vi "supermlo photo v3_LV2010 GFIREST VARIANT.vi"() -> ()   [LabVIEW 2010]
uses:
  <vilib>/Utility/file.llb/Read From Spreadsheet File (DBL).vi
  Instance          10 25Saved   supermlo photo v3 .vi
  Instance           9 25Saved   supermlo photo v3 .vi
  Instance           8 25Saved   supermlo photo v3 .vi
  Instance          15 25Saved   supermlo photo v3 .vi
  Instance          16 25Saved   supermlo photo v3 .vi
  Instance          17 25Saved   supermlo photo v3 .vi
  Instance          12 25Saved   supermlo photo v3 .vi
  Instance          13 25Saved   supermlo photo v3 .vi
  Instance          14 25Saved   supermlo photo v3 .vi
  <vilib>/Utility/file.llb/Write To Spreadsheet File (DBL).vi
panel:
  out "Lockin corrected counter graoh":cluster{"all rows":dbl[], "all rows":dbl[]}[](graph)
  in  "Lockin panel":T1={"slope"=1, "Input Mode"=0, "time constant"=6, "display type"=1, "Range"=7, "Line reject"=1, "Filter Type"=0, "Auto freq tuning"=TRUE, "Filter Frequency (Hz)"=1000.0, "Auto Sensitivity"=FALSE, "Auto Measure"=FALSE, "Auto Phase"=TRUE} {"Filter Frequency (Hz)" min=2.0 max=1250000.0 step=1.0; "Filter Type" items=["Flat", "Notch", "Low-Pass", "Bandpass"]; "Line reject" items=["OFF", "2F", "F", "F & 2F"]; "Range" items=["100 nV", "300 nV", "1 uV", "3 uV", "10 uV", "30 uV", "100 uV", "300 uV", "1 mV", "3 mV", "10 mV", "30 mV", "100 mV", "300 mV", "1 V", "3 V"]; "display type" items=["Output %", "Output calibrated ", "Ratio", "log Ratio", "ADC 1", "ADC 2", " ADC 3", "ADC 4", "Noise %", "Noise Calibrated", "Ref. Frequency"]; "time constant" items=["1 ms", "3 ms", "10 ms", "30 ms", "100 ms", "300 ms", "1 s", "3 s", "10 s", "30 s", "100 s", "300 s", "1 ks", "3 ks"]; "Input Mode" items=["Voltage Input ( A or A-B)", "Current Input 10E6 V/A", "Current Input 10E8 V/A"]; "slope" items=["6dB/octave", "12dB/octave"]}
  out "Wavelength Range Warning":bool
  out "wavelength":i32=692
  out "counter A":i32=70
  out "counter B":i32
  out "lockin":dbl=78.0 format="%.3e"
  out "Lockin Graph":cluster{"all rows":dbl[], "all rows":dbl[]}[](graph)
  out "Counter Graph":cluster{"all rows":dbl[], "all rows":dbl[]}[](graph)
  in  "GPIB Address Lock-In":u8=12 min=1 max=32 step=1
  in  "GPIB Address OSC (GPIB::4)":string="GPIB0::4"
  in  "Parallel Port Address":i16=888 format="%.0x"
  in  "Mode Control":T2(tab)=enum."Sweep 2"
  in  "Wavelength":dbl=500.0
  out "Waveform Graph":cluster{ext, ext, ext[]}(graph)
  in  "Pull Data From Oscilloscope":bool
  in  "waveform source (ch1:0)":i32(ring) items=["Channel 1", "Channel 2", "Channel 3", "Channel 4", "Reference 1", "Reference 2", "Reference 3", "Reference 4", "Math 1", "Math 2", "Math 3"]
  in  "Time For Scan (seconds)":dbl=30.0
  in  "Final Wavelength (scan)":dbl=425.0
  in  "Initial Wavelength (scan)":dbl=546.0
  out "XY Graph":cluster{"Y":dbl[], "Y":dbl[]}[](graph)=[{"Y"=[424.0, 425.0, 426.0, 427.0, 428.0, 429.0, 430.0, 431.0, 432.0, 433.0, 434.0], "Y"=[23.190000534057617, 23.65999984741211, 23.200000762939453, 22.600000381469727, 24.850000381469727, 24.90999984741211, 24.979999542236328, 24.940000534057617, 24.829999923706055, 24.860000610351562, 24.799999237060547]}]
  in  "Wait Time (s)":dbl=50.0
  in  "Step Size (nm)":dbl=1.0
  in  "Final Wavelength (sweep)":dbl=435.0
  in  "Initial Wavelength (sweep)":dbl=424.0
  in  "raster settings\nxV xHz yV yHz":string
  in  "note":string
  in  "532 power":string="0"
  in  "Green Filter in = 1":string="1"
  out "String":string
  in  "Wait Time (s) (sweep2)":dbl=5.0
  in  "Step Size (nm) (sweep2)":dbl=1.0
  in  "Final Wavelength (sweep2)":dbl=510.0
  in  "Initial Wavelength (sweep2)":dbl=420.0
  in  "Start Wavelength":dbl=430.0
  # "Oscilloscope Setup"
  # "Monochromator Setup"
  # "Lock-In Setup"
  # "GABE'S VARIANT, appends to TEMP rather than overwrites"
  # "LAST DATA POINT"
  # "Lockin Amplifier"
  # "SR400 photon counter:\n1. Run photon counter vi\nor manually control desired\nsettings.\n2. Set Wait Time to Tpreset\n3. Run this program.\nnote: # count periods N = 1"
  # "Note: set wait time to\nTpreset value on SR400"
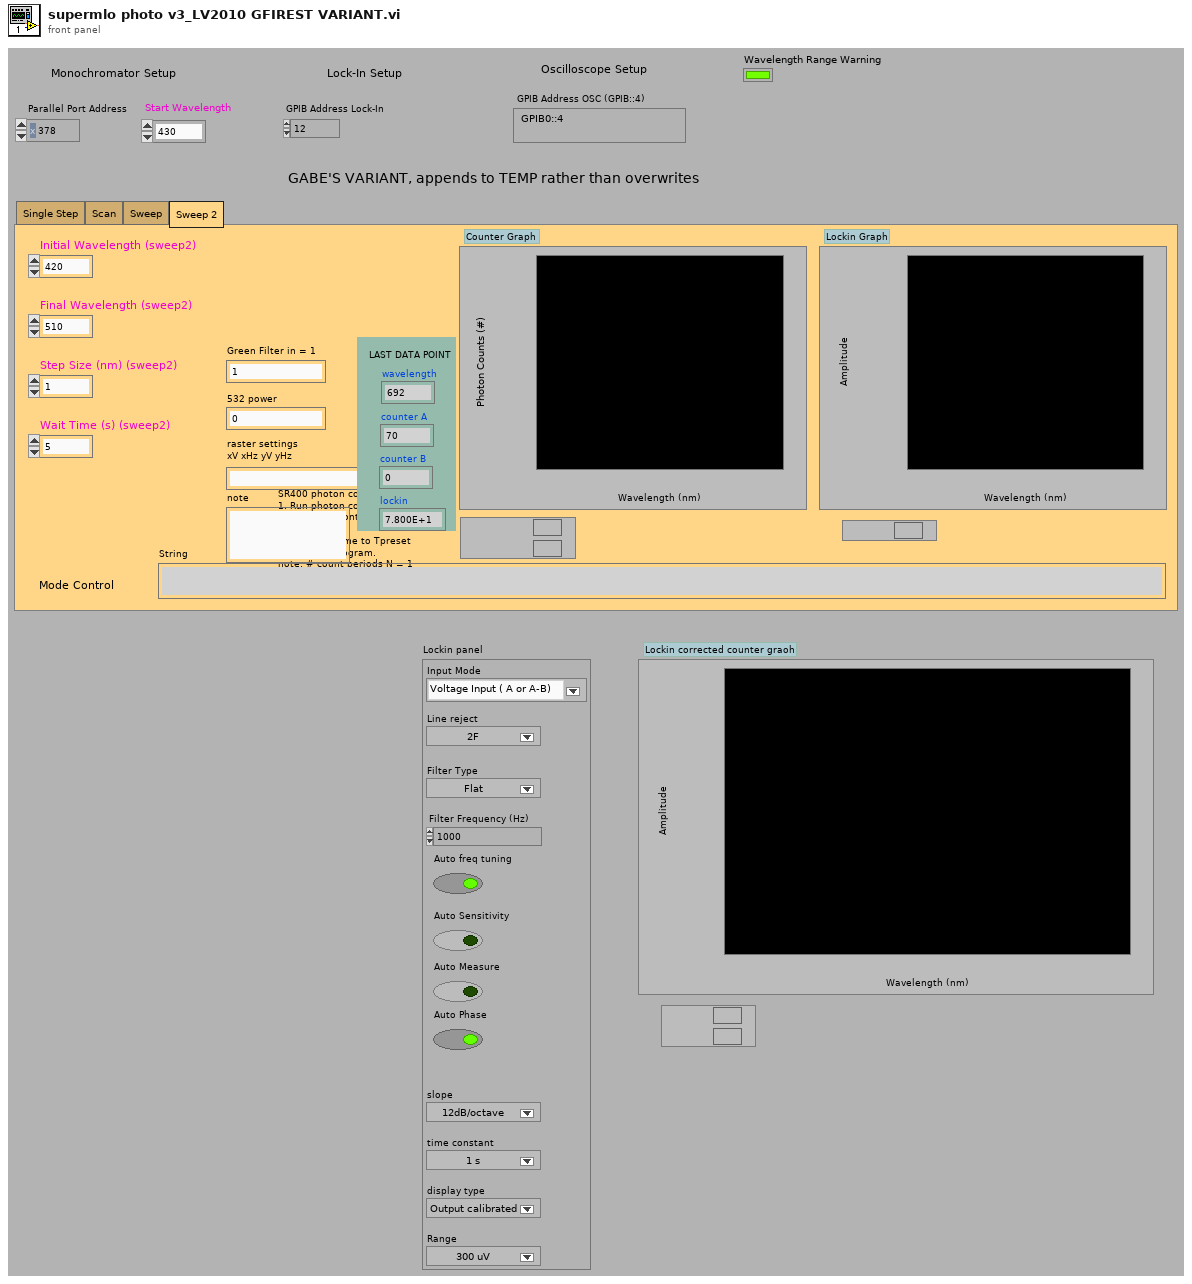
[diagram p1: front panel]
types:
  T1 = cluster{"slope":i32, "Input Mode":i32, "time constant":i32, "display type":i32, "Range":i32, "Line reject":i32, "Filter Type":i32, "Auto freq tuning":bool, "Filter Frequency (Hz)":dbl, "Auto Sensitivity":bool, "Auto Measure":bool, "Auto Phase":bool}
  T2 = enum32{"Single Step", "Scan", "Sweep", "Sweep 2"}
  T3 = enum16{"open", "open or create", "create or replace", "create", "open (read only)"}
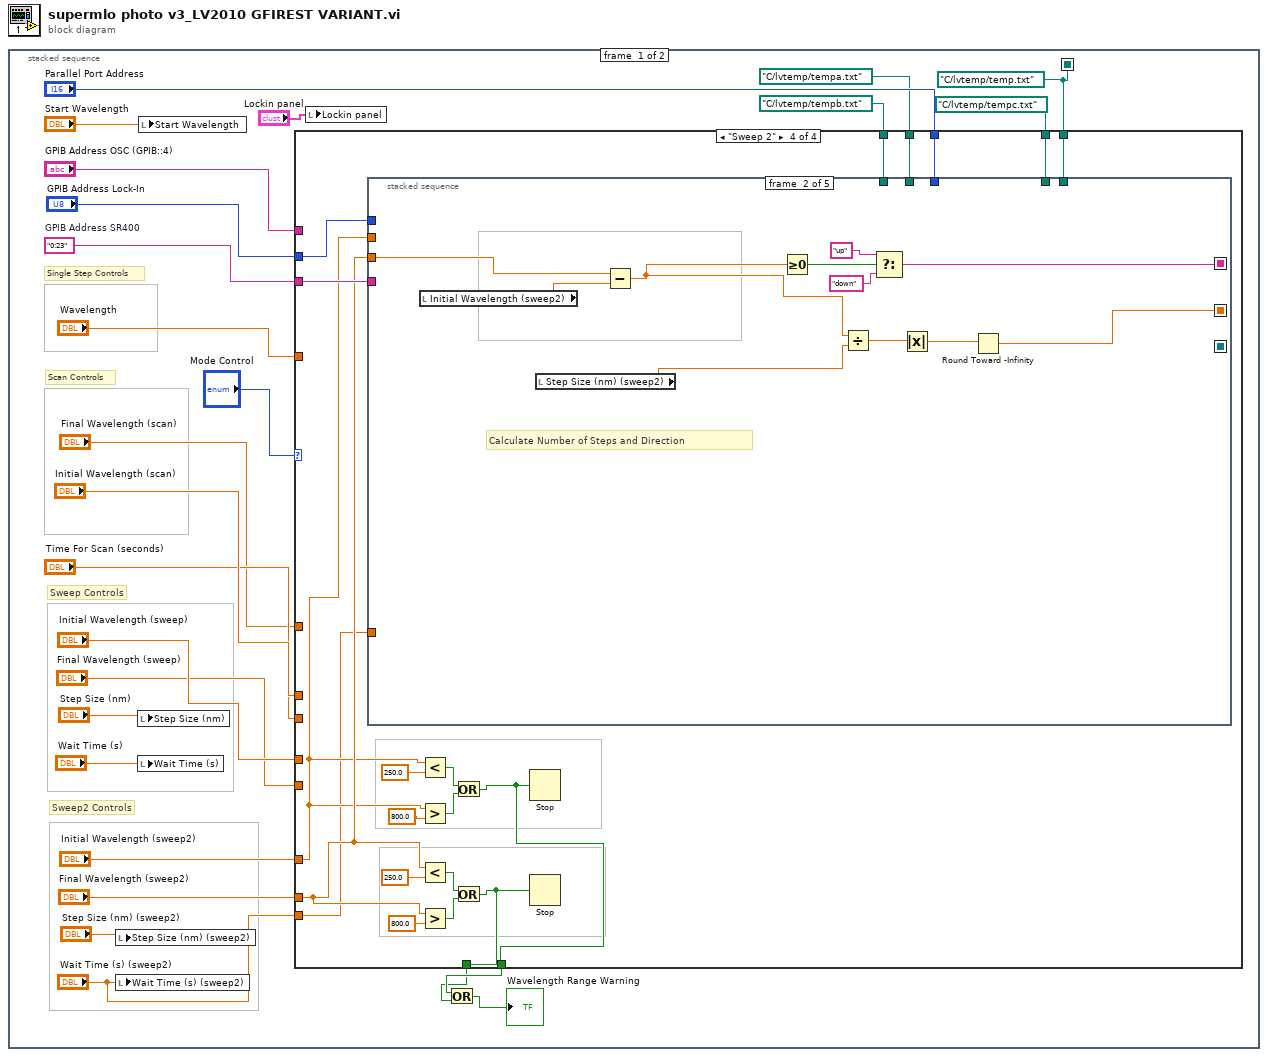
[diagram p0: block diagram]
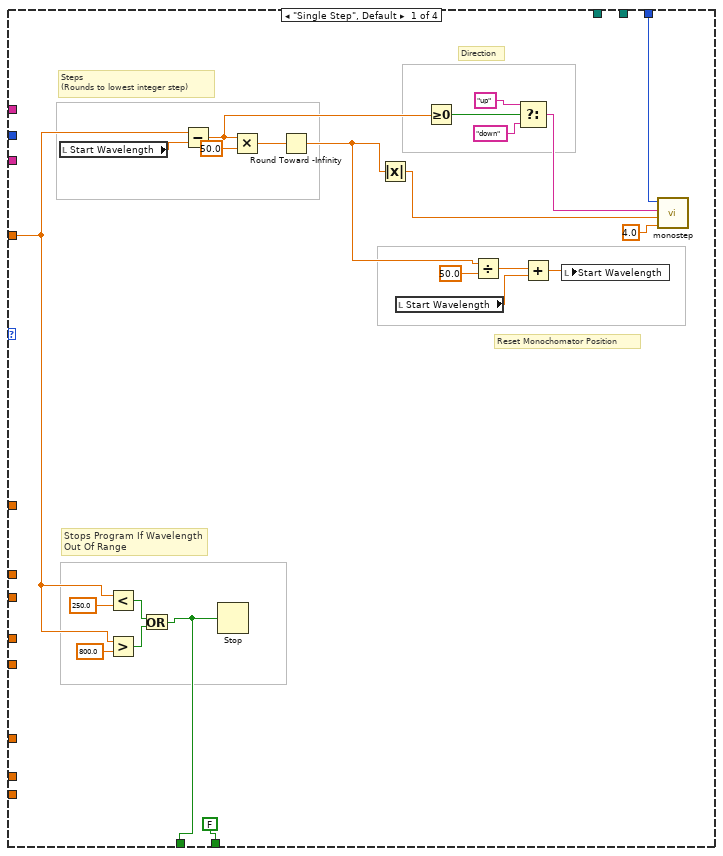
[diagram p2: hidden frame]
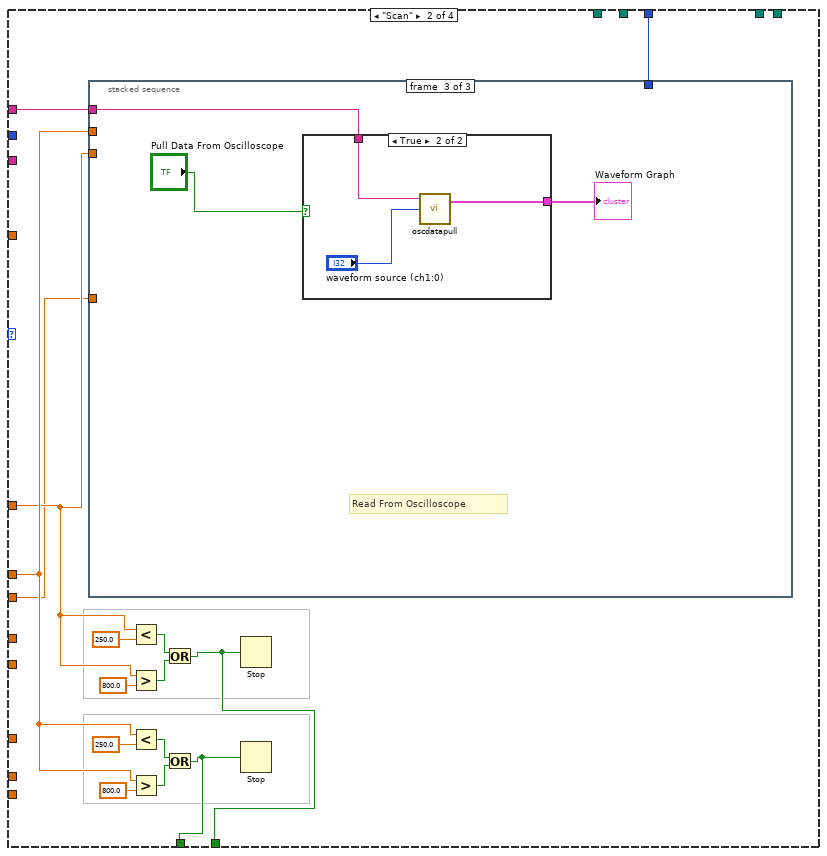
[diagram p3: hidden frame]
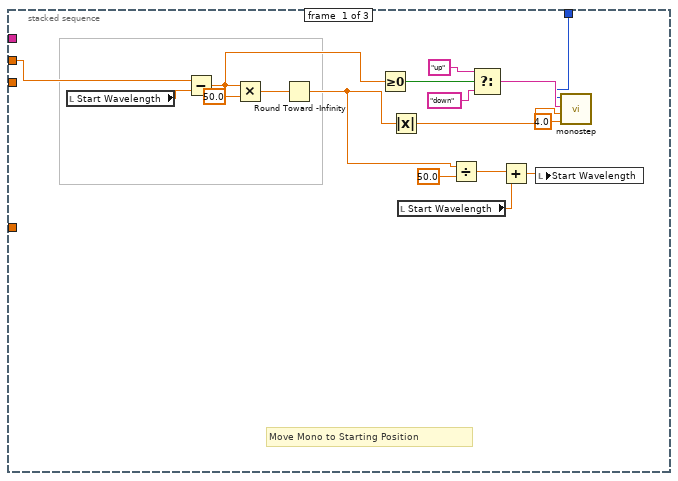
[diagram p4: hidden frame]
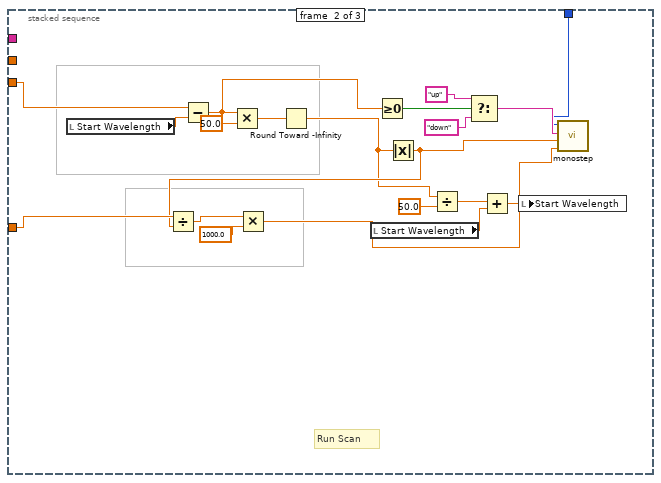
[diagram p5: hidden frame]
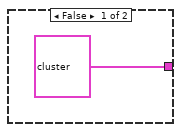
[diagram p6: hidden frame]
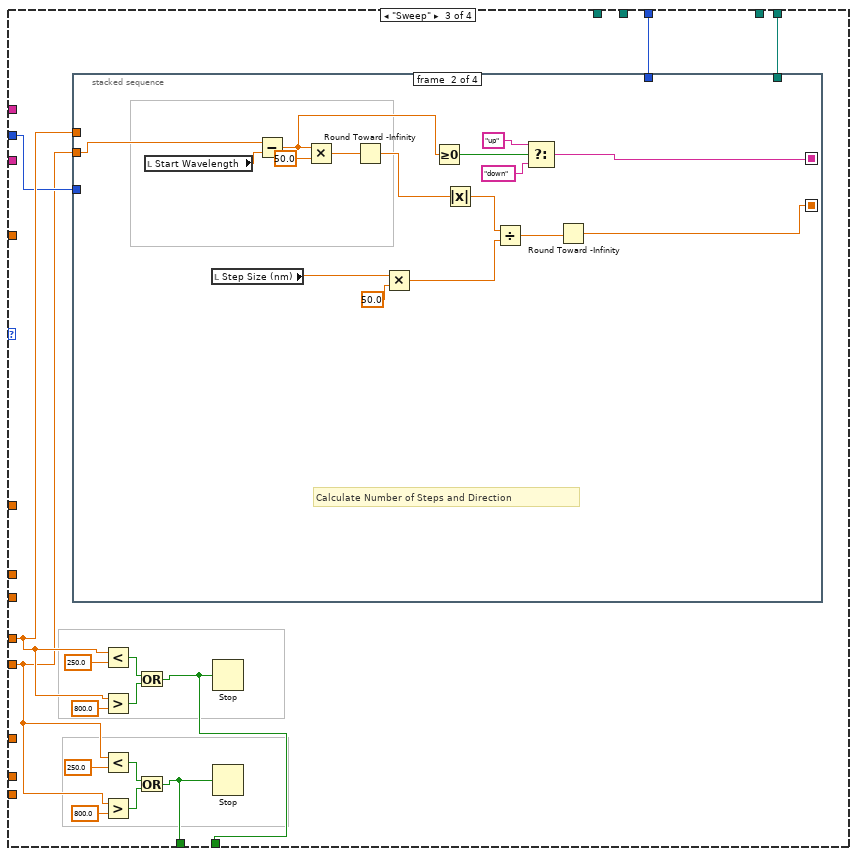
[diagram p7: hidden frame]
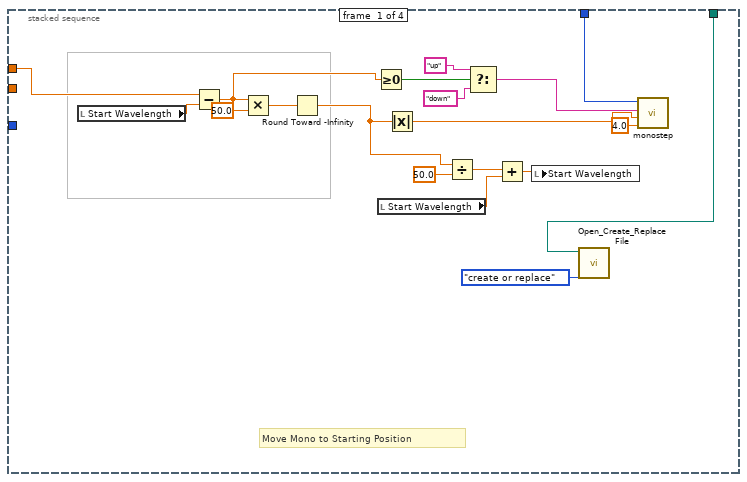
[diagram p8: hidden frame]
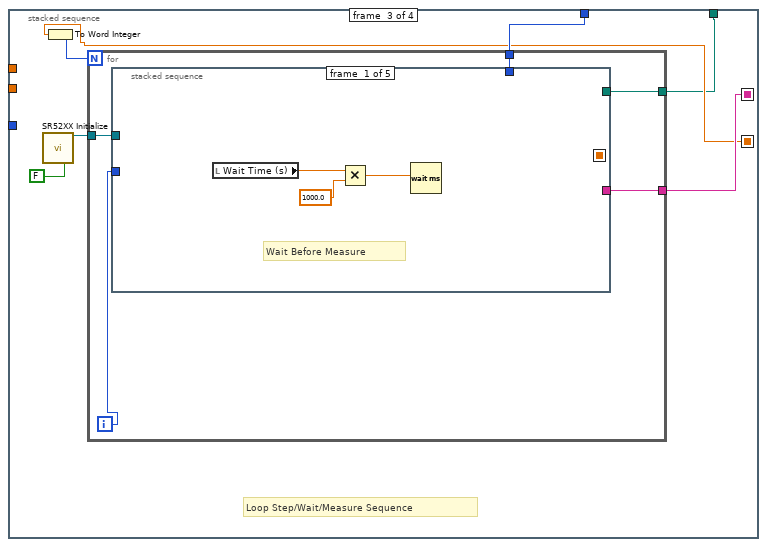
[diagram p9: hidden frame]
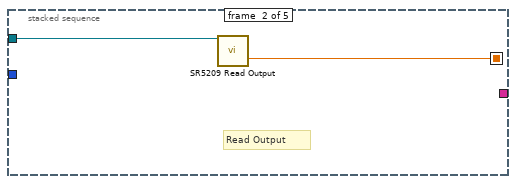
[diagram p10: hidden frame]
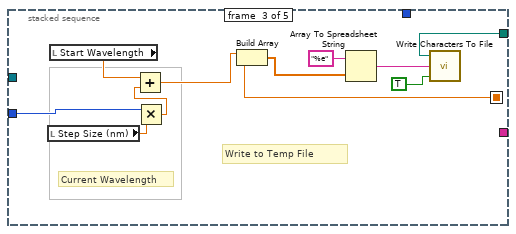
[diagram p11: hidden frame]
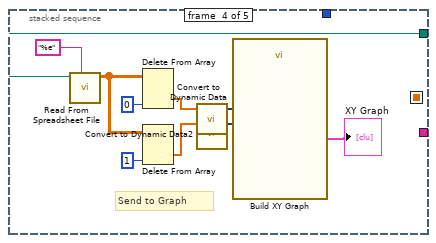
[diagram p12: hidden frame]
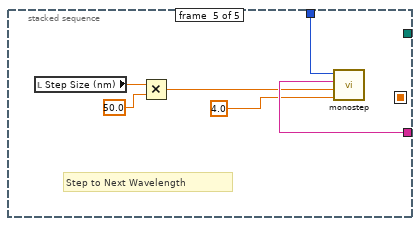
[diagram p13: hidden frame]
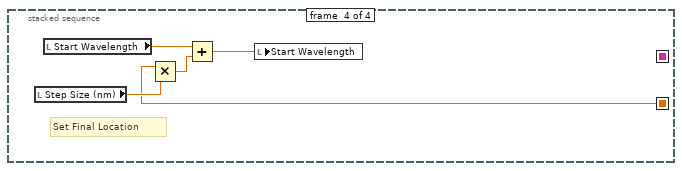
[diagram p14: hidden frame]
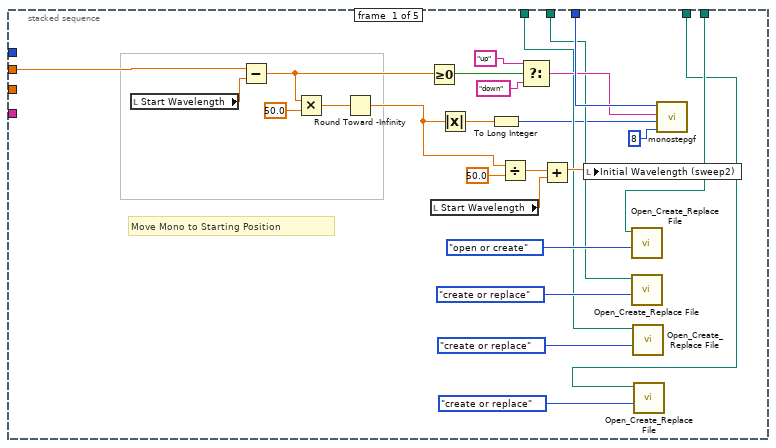
[diagram p15: hidden frame]
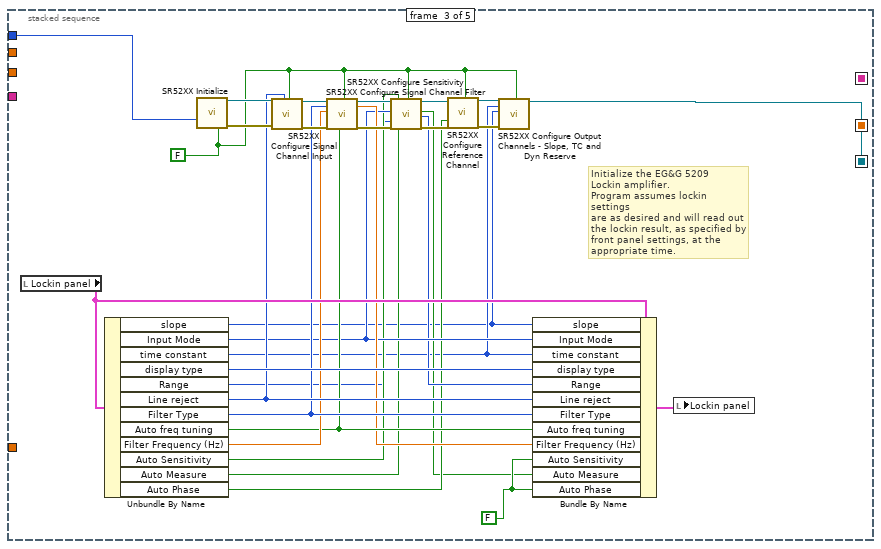
[diagram p16: hidden frame]
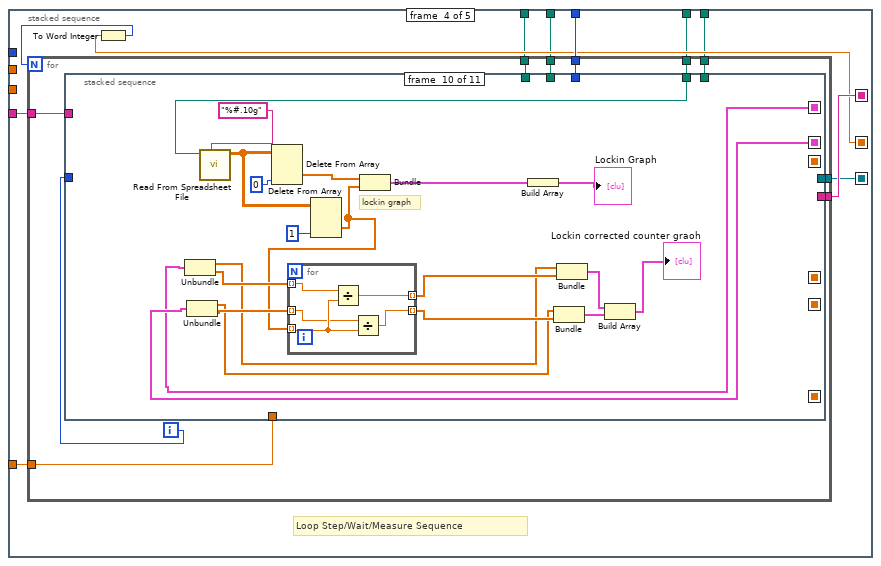
[diagram p17: hidden frame]
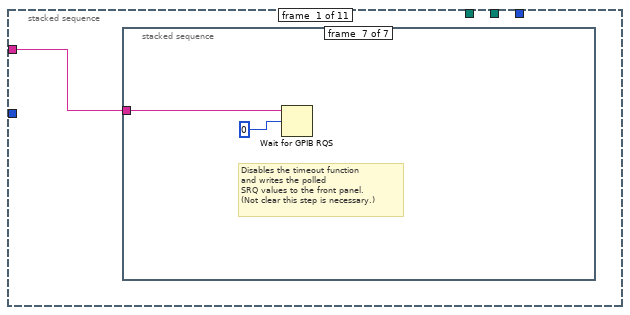
[diagram p18: hidden frame]
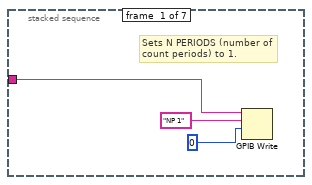
[diagram p19: hidden frame]
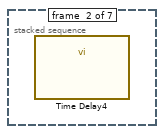
[diagram p20: hidden frame]
diagram:
  n1 = stacked-sequence {
    seq-local: [w6 _] -> [_ w468]
    frame #0 {
      w6 = path "C:/lvtemp/temp.txt" ("file path")
      w13 = "0:23"  # GPIB Address SR400
      # "Sweep2 Controls"
      # "Sweep Controls"
      # "Scan Controls"
      # "Single Step Controls"
      n2 = local write "Step Size (nm) (sweep2)"("Step Size (nm) (sweep2)") -> ()
      n3 = local write "Wait Time (s) (sweep2)"("Wait Time (s) (sweep2)") -> ()
      n4 = local write "Step Size (nm)"("Step Size (nm)") -> ()
      n5 = local write "Wait Time (s)"("Wait Time (s)") -> ()
      n6 = local write "Start Wavelength"("Start Wavelength") -> ()
      n7 = case shown="\"Sweep 2\"" "Mode Control" {
        tunnel: "Wavelength" -> [w42 _ _ _]
        tunnel: "Parallel Port Address" -> [w36 w56 w112 w217]
        tunnel: "Final Wavelength (scan)" -> [_ w54 _ _]
        tunnel: "Initial Wavelength (scan)" -> [_ w55 _ _]
        tunnel: "Time For Scan (seconds)" -> [_ w53 _ _]
        tunnel: "GPIB Address OSC (GPIB::4)" -> [_ w52 _ _]
        tunnel: [FALSE w51 w115 w219] -> w20
        tunnel: [w30 w50 w114 w218] -> w19
        tunnel: "Initial Wavelength (sweep)" -> [_ _ w113 _]
        tunnel: "Final Wavelength (sweep)" -> [_ _ w110 _]
        tunnel: "GPIB Address Lock-In" -> [_ _ w111 w210]
        tunnel: w13 -> [_ _ _ w216]
        tunnel: "Final Wavelength (sweep2)" -> [_ _ _ w215]
        tunnel: "Initial Wavelength (sweep2)" -> [_ _ _ w214]
        tunnel: w6 -> [_ _ w109 w213]
        tunnel: path "C:/lvtemp/tempa.txt" ("file path") -> [_ _ _ w212]
        tunnel: path "C:/lvtemp/tempb.txt" ("file path") -> [_ _ _ w211]
        tunnel: path "C:/lvtemp/tempc.txt" ("file path") -> [_ _ _ w209]
        tunnel: "Wait Time (s) (sweep2)" -> [_ _ _ w208]
        frame "Single Step", Default {
          # "Reset Monochomator Position"
          # "Direction"
          # "Stops Program If Wavelength\nOut Of Range"
          # "Steps \n(Rounds to lowest integer step)"
          n8 = local read "Start Wavelength"() -> (w47:dbl)
          n9 = Less?(x=w42, y=250.0) -> (x < y?=w44:bool)
          n10 = Greater?(x=w42, y=800.0) -> (0:w43:bool)
          n11 = Or(x=w44, y=w43) -> (x .or. y?=w30:bool)
          n12 = Subtract(x=w42, y=w47) -> (x-y=w37:dbl)
          n13 = Stop(stop? (T)=w30) -> ()
          n14 = Multiply(x=w37, y=50.0) -> (x*y=w48:dbl)
          n15 = Round Toward -Infinity(1:w48) -> (0:w28:dbl)
          n16 = Absolute Value(x=w28) -> (abs(x)=w33:dbl)
          n17 = local read "Start Wavelength"() -> (w32:dbl)
          n18 = Greater Or Equal To 0?(x=w37) -> (x >= 0?=w41:bool)
          n19 = Divide(x=w28, y=50.0) -> (x/y=w34:dbl)
          n20 = Select(t="up", s=w41, f="down") -> (s? t:f=w38:string)
          n21 = Add(x=w34, y=w32) -> (x+y=w31:dbl)
          n22 = local write "Start Wavelength"(w31) -> ()
          n23 = call "monostep.vi"("Wait Between Steps(ms)"=4.0, "Steps"=w33, "Direction"=w38, "address"=w36) -> ()
        }
        frame "Scan" {
          n24 = stacked-sequence {
            tunnel: w56 -> [w76 w94 _]
            tunnel: w55 -> [w71 _ _]
            tunnel: w54 -> [_ w93 _]
            tunnel: w53 -> [_ w87 _]
            tunnel: w52 -> [_ _ w103]
            frame #0 {
              # "Move Mono to Starting Position"
              n25 = local read "Start Wavelength"() -> (w72:dbl)
              n26 = Subtract(x=w71, y=w72) -> (x-y=w73:dbl)
              n27 = Multiply(x=w73, y=50.0) -> (x*y=w74:dbl)
              n28 = Round Toward -Infinity(1:w74) -> (0:w65:dbl)
              n29 = Greater Or Equal To 0?(x=w73) -> (x >= 0?=w81:bool)
              n30 = Absolute Value(x=w65) -> (abs(x)=w70:dbl)
              n31 = local read "Start Wavelength"() -> (w68:dbl)
              n32 = Divide(x=w65, y=50.0) -> (x/y=w67:dbl)
              n33 = Select(t="up", s=w81, f="down") -> (s? t:f=w78:string)
              n34 = Add(x=w67, y=w68) -> (x+y=w66:dbl)
              n35 = local write "Start Wavelength"(w66) -> ()
              n36 = call "monostep.vi"("Wait Between Steps(ms)"=4.0, "Steps"=w70, "Direction"=w78, "address"=w76) -> ()
            }
            frame #1 {
              # "Run Scan"
              n37 = local read "Start Wavelength"() -> (w92:dbl)
              n38 = Subtract(x=w93, y=w92) -> (x-y=w95:dbl)
              n39 = Multiply(x=w95, y=50.0) -> (x*y=w96:dbl)
              n40 = Round Toward -Infinity(1:w96) -> (0:w82:dbl)
              n41 = local read "Start Wavelength"() -> (w89:dbl)
              n42 = Greater Or Equal To 0?(x=w95) -> (x >= 0?=w101:bool)
              n43 = Absolute Value(x=w82) -> (abs(x)=w86:dbl)
              n44 = Divide(x=w87, y=w86) -> (x/y=w85:dbl)
              n45 = Multiply(x=w85, y=1000.0) -> (x*y=w83:dbl)
              n46 = Divide(x=w82, y=50.0) -> (x/y=w90:dbl)
              n47 = Select(t="up", s=w101, f="down") -> (s? t:f=w98:string)
              n48 = Add(x=w90, y=w89) -> (x+y=w88:dbl)
              n49 = local write "Start Wavelength"(w88) -> ()
              n50 = call "monostep.vi"("Wait Between Steps(ms)"=w83, "Steps"=w86, "Direction"=w98, "address"=w94) -> ()
            }
            frame #2 {
              # "Read From Oscilloscope"
              n51 = case shown="True" "Pull Data From Oscilloscope" {
                tunnel: w103 -> [_ w108]
                tunnel: [cluster{ext, ext, ext[]} {0.0, 0.0, []} ("returned waveform") w106] -> w102
                frame False {
                }
                frame True {
                  n52 = call "oscdatapull.vi"("waveform source (ch1:0)"="waveform source (ch1:0)", "instrument descriptor (GPIB::4)"=w108) -> ("returned waveform"=w106:cluster{ext, ext, ext[]})  [unwired: 2 in]
                }
              }
              "Waveform Graph" <- w102
            }
          }
          n53 = Less?(x=w54, y=250.0) -> (x < y?=w62:bool)
          n54 = Greater?(x=w54, y=800.0) -> (0:w61:bool)
          n55 = Less?(x=w55, y=250.0) -> (x < y?=w58:bool)
          n56 = Greater?(x=w55, y=800.0) -> (0:w57:bool)
          n57 = Or(x=w62, y=w61) -> (x .or. y?=w51:bool)
          n58 = Or(x=w58, y=w57) -> (x .or. y?=w50:bool)
          n59 = Stop(stop? (T)=w51) -> ()
          n60 = Stop(stop? (T)=w50) -> ()
        }
        frame "Sweep" {
          n61 = stacked-sequence {
            seq-local: [_ w150 _ _] -> [_ _ w162 _]
            seq-local: [_ w145 _ _] -> [_ _ w161 w205]
            tunnel: w113 -> [w133 _ _ _]
            tunnel: w112 -> [w129 _ w163 _]
            tunnel: w111 -> [_ _ _ _]
            tunnel: w110 -> [_ w144 _ _]
            tunnel: w109 -> [w124 _ w159 _]
            frame #0 {
              # "Move Mono to Starting Position"
              n62 = local read "Start Wavelength"() -> (w134:dbl)
              n63 = Subtract(x=w133, y=w134) -> (x-y=w132:dbl)
              n64 = Multiply(x=w132, y=50.0) -> (x*y=w141:dbl)
              n65 = Round Toward -Infinity(1:w141) -> (0:w125:dbl)
              n66 = Greater Or Equal To 0?(x=w132) -> (x >= 0?=w140:bool)
              n67 = local read "Start Wavelength"() -> (w131:dbl)
              n68 = Absolute Value(x=w125) -> (abs(x)=w127:dbl)
              n69 = Divide(x=w125, y=50.0) -> (x/y=w136:dbl)
              n70 = Select(t="up", s=w140, f="down") -> (s? t:f=w128:string)
              n71 = Add(x=w136, y=w131) -> (x+y=w130:dbl)
              n72 = local write "Start Wavelength"(w130) -> ()
              n73 = call <vilib>:"Open_Create_Replace File.vi"("function (open:0)"=T3."create or replace", "file path"=w124) -> ()  [unwired: 6 in, 4 out]
              n74 = call "monostep.vi"("Wait Between Steps(ms)"=4.0, "Steps"=w127, "Direction"=w128, "address"=w129) -> ()
            }
            frame #1 {
              # "Calculate Number of Steps and Direction"
              n75 = local read "Start Wavelength"() -> (w156:dbl)
              n76 = local read "Step Size (nm)"() -> (w143:dbl)
              n77 = Subtract(x=w144, y=w156) -> (x-y=w152:dbl)
              n78 = Multiply(x=w152, y=50.0) -> (x*y=w157:dbl)
              n79 = Round Toward -Infinity(1:w157) -> (0:w151:dbl)
              n80 = Multiply(x=w143, y=50.0) -> (x*y=w147:dbl)
              n81 = Greater Or Equal To 0?(x=w152) -> (x >= 0?=w155:bool)
              n82 = Absolute Value(x=w151) -> (abs(x)=w148:dbl)
              n83 = Divide(x=w148, y=w147) -> (x/y=w146:dbl)
              n84 = Select(t="up", s=w155, f="down") -> (s? t:f=w150:string)
              n85 = Round Toward -Infinity(1:w146) -> (0:w145:dbl)
            }
            frame #2 {
              # "Loop Step/Wait/Measure Sequence"
              n86 = call "SR52XX Initialize"("reset"=FALSE) -> ("VISA session"=w164:refnum<visa-resource-name>)  [unwired: 12 in, 2 out]
              n87 = To Word Integer(number=w161) -> (16bit integer=w160:i16)
              n88 = for {
                N: w160 -> [_]
                tunnel: w164 -> [w170]
                tunnel: w163 -> [w168]
                tunnel: w162 -> [w167]
                tunnel: w159 -> [w166]
                i -> [w169]
                n89 = stacked-sequence {
                  seq-local: [_ w174 _ _ _] -> [_ _ w181 _ _]
                  tunnel: w170 -> [_ w175 _ _ _]
                  tunnel: w169 -> [_ _ w185 _ _]
                  tunnel: w168 -> [_ _ _ _ w197]
                  tunnel: w167 -> [_ _ _ _ w202]
                  tunnel: w166 -> [_ _ w176 w187 _]
                  frame #0 {
                    # "Wait Before Measure"
                    n90 = local read "Wait Time (s)"() -> (w173:dbl)
                    n91 = Multiply(x=w173, y=1000.0) -> (x*y=w171:dbl)
                    n92 = Wait (ms)(milliseconds to wait=w171) -> ()  [unwired: 1 out]
                  }
                  frame #1 {
                    # "Read Output"
                    n93 = call "SR5209 Read Output"("VISA session (for class)"=w175) -> ("Output (FP)"=w174:dbl)  [unwired: 10 in, 8 out]
                  }
                  frame #2 {
                    # "Write to Temp File"
                    # "Current Wavelength"
                    n94 = local read "Step Size (nm)"() -> (w184:dbl)
                    n95 = local read "Start Wavelength"() -> (w186:dbl)
                    n96 = Multiply(x=w185, y=w184) -> (x*y=w183:dbl)
                    n97 = Add(x=w186, y=w183) -> (x+y=w182:dbl)
                    n98 = Build Array(w182, w181) -> (w178:dbl[])
                    n99 = Array To Spreadsheet String(array=w178, 3:"%e" ("format string")) -> (spreadsheet string=w177:string)  [unwired: 1 in]
                    n100 = call <vilib>:"Write Characters To File.vi"("append to file? (new file:F)"=TRUE, "character string"=w177, "file path (dialog if empty)"=w176) -> ()  [unwired: 2 in, 1 out]
                  }
                  frame #3 {
                    # "Send to Graph"
                    n101 = call-poly <vilib>:"Read From Spreadsheet File.vi"("format (%.3f)"="%e", "file path (dialog if empty)"=w187) -> ("all rows"=w193:dbl[][])  [unwired: 5 in, 4 out]
                    n102 = Delete From Array(array=w193, index (col)=0 ("disabled index (col)")) -> (deleted portion=w191:dbl[])  [unwired: 2 in, 1 out]
                    n103 = Delete From Array(array=w193, index (col)=1 ("disabled index (col)")) -> (deleted portion=w189:dbl[])  [unwired: 2 in, 1 out]
                    n104 = call "Convert to Dynamic Data"("Array"=w191) -> ("Dynamic Data Type"=w190:dynamicdata)  [unwired: 3 in]
                    n105 = call "Convert to Dynamic Data2"("Array"=w189) -> ("Dynamic Data Type"=w188:dynamicdata)  [unwired: 3 in]
                    n106 = call "Build XY Graph"("Y Input"=w188, "X Input"=w190) -> ("XY Graph"=→"XY Graph":cluster{"Y":dbl[], "Y":dbl[]}[])  [unwired: 8 in, 1 out]
                  }
                  frame #4 {
                    # "Step to Next Wavelength"
                    n107 = local read "Step Size (nm)"() -> (w201:dbl)
                    n108 = Multiply(x=w201, y=50.0) -> (x*y=w199:dbl)
                    n109 = call "monostep.vi"("Wait Between Steps(ms)"=4.0, "Steps"=w199, "Direction"=w202, "address"=w197) -> ()
                  }
                }
              }
            }
            frame #3 {
              # "Set Final Location"
              n110 = local read "Step Size (nm)"() -> (w206:dbl)
              n111 = local read "Start Wavelength"() -> (w207:dbl)
              n112 = Multiply(x=w205, y=w206) -> (x*y=w204:dbl)
              n113 = Add(x=w207, y=w204) -> (x+y=w203:dbl)
              n114 = local write "Start Wavelength"(w203) -> ()
            }
          }
          n115 = Less?(x=w113, y=250.0) -> (x < y?=w121:bool)
          n116 = Greater?(x=w113, y=800.0) -> (0:w120:bool)
          n117 = Less?(x=w110, y=250.0) -> (x < y?=w117:bool)
          n118 = Greater?(x=w110, y=800.0) -> (0:w116:bool)
          n119 = Or(x=w121, y=w120) -> (x .or. y?=w115:bool)
          n120 = Or(x=w117, y=w116) -> (x .or. y?=w114:bool)
          n121 = Stop(stop? (T)=w115) -> ()
          n122 = Stop(stop? (T)=w114) -> ()
        }
        frame "Sweep 2" {
          n123 = stacked-sequence {
            seq-local: [_ w260 _ _ _] -> [_ _ _ w305 _]
            seq-local: [_ w254 _ _ _] -> [_ _ _ w304 w464]
            seq-local: [_ _ w285 _ _] -> [_ _ _ w298 _]
            tunnel: w214 -> [w244 _ _ _ _]
            tunnel: w217 -> [w240 _ _ w306 w450]
            tunnel: w215 -> [_ w259 _ _ _]
            tunnel: w216 -> [_ _ _ w302 _]
            tunnel: w213 -> [w235 _ _ w301 _]
            tunnel: w212 -> [w234 _ _ w300 _]
            tunnel: w211 -> [w231 _ _ w299 _]
            tunnel: w210 -> [_ _ w295 _ _]
            tunnel: w209 -> [w229 _ _ w297 _]
            tunnel: w208 -> [_ _ _ w296 _]
            frame #0 {
              # "Move Mono to Starting Position"
              n124 = local read "Start Wavelength"() -> (w245:dbl)
              n125 = Subtract(x=w244, y=w245) -> (x-y=w243:dbl)
              n126 = Multiply(x=w243, y=50.0) -> (x*y=w252:dbl)
              n127 = Round Toward -Infinity(1:w252) -> (0:w236:dbl)
              n128 = Greater Or Equal To 0?(x=w243) -> (x >= 0?=w251:bool)
              n129 = local read "Start Wavelength"() -> (w242:dbl)
              n130 = Absolute Value(x=w236) -> (abs(x)=w238:dbl)
              n131 = To Long Integer(number=w238) -> (32bit integer=w228:i32)
              n132 = Divide(x=w236, y=50.0) -> (x/y=w247:dbl)
              n133 = Select(t="up", s=w251, f="down") -> (s? t:f=w239:string)
              n134 = Add(x=w247, y=w242) -> (x+y=w241:dbl)
              n135 = local write "Initial Wavelength (sweep2)"(w241) -> ()
              n136 = call <vilib>:"Open_Create_Replace File.vi"("function (open:0)"=T3."open or create", "file path"=w235) -> ()  [unwired: 6 in, 4 out]
              n137 = call <vilib>:"Open_Create_Replace File.vi"("function (open:0)"=T3."create or replace", "file path"=w234) -> ()  [unwired: 6 in, 4 out]
              n138 = call <vilib>:"Open_Create_Replace File.vi"("function (open:0)"=T3."create or replace", "file path"=w231) -> ()  [unwired: 6 in, 4 out]
              n139 = call <vilib>:"Open_Create_Replace File.vi"("function (open:0)"=T3."create or replace", "file path"=w229) -> ()  [unwired: 6 in, 4 out]
              n140 = call "monostepgf.vi"("Wait Between Steps(ms)"=u32 8, "Steps"=w228, "Direction"=w239, "address"=w240) -> ()
            }
            frame #1 {
              # "Calculate Number of Steps and Direction"
              n141 = local read "Initial Wavelength (sweep2)"() -> (w264:dbl)
              n142 = local read "Step Size (nm) (sweep2)"() -> (w257:dbl)
              n143 = Subtract(x=w259, y=w264) -> (x-y=w258:dbl)
              n144 = Greater Or Equal To 0?(x=w258) -> (x >= 0?=w263:bool)
              n145 = Divide(x=w258, y=w257) -> (x/y=w256:dbl)
              n146 = Select(t="up", s=w263, f="down") -> (s? t:f=w260:string)
              n147 = Absolute Value(x=w256) -> (abs(x)=w255:dbl)
              n148 = Round Toward -Infinity(1:w255) -> (0:w254:dbl)
            }
            frame #2 {
              w281 = FALSE ("reset")
              w283 = FALSE ("reset")
              # "Initialize the EG&G 5209\nLockin amplifier.\nProgram assumes lockin settings\nare as desired and will read out\nthe lockin result, as specified by \nfront panel settings, at the\nappropriate time."
              n149 = local read "Lockin panel"() -> (w279:T1)
              n150 = Unbundle By Name(w279) -> ("slope"=w265:i32, "Input Mode"=w273:i32, "time constant"=w266:i32, "display type"=w282:i32, "Range"=w271:i32, "Line reject"=w278:i32, "Filter Type"=w277:i32, "Auto freq tuning"=w275:bool, "Filter Frequency (Hz)"=w276:dbl, "Auto Sensitivity"=w272:bool, "Auto Measure"=w270:bool, "Auto Phase"=w268:bool)
              n151 = call "SR52XX Initialize"("Port"=w295, "reset"=w283) -> ("VISA session"=w286:refnum<visa-resource-name>, "error out"=w284:errorcluster)  [unwired: 11 in, 1 out]
              n152 = call "SR52XX Configure Signal Channel Input"("VISA session (for class)"=w286, "error in (no error)"=w284, "Line Frequency Rejection Filter"=w278, "Update"=w283) -> ("VISA session"=w294:refnum<visa-resource-name>, "error out"=w292:errorcluster)  [unwired: 14 in]
              n153 = call "SR52XX Configure Signal Channel Filter"("VISA session (for class)"=w294, "FilterType"=w277, "Filter Frequency (Hz)"=w276, "error in (no error)"=w292, "Filter Tuning"=w275, "Update"=w283) -> ("VISA session"=w293:refnum<visa-resource-name>, "Filter Frequency (Hz) out"=w274:dbl, "error out"=w291:errorcluster)  [unwired: 11 in]
              n154 = call "SR52XX Configure Sensitivity"("VISA session (for class)"=w293, "Input Mode"=w273, "Range"=w271, "error in (no error)"=w291, "Auto Sensitivity"=w272, "Auto Measure"=w270, "Update"=w283) -> ("VISA session"=w290:refnum<visa-resource-name>, "Auto Measure out"=w267:bool, "Range Out"=w269:u8, "error out"=w289:errorcluster)  [unwired: 7 in, 2 out]
              n155 = call "SR52XX Configure Reference Channel"("VISA session (for class)"=w290, "Auto Phase"=w268, "error in (no error)"=w289, "Update"=w283) -> ("VISA session"=w288:refnum<visa-resource-name>, "error out"=w287:errorcluster)  [unwired: 12 in, 2 out]
              n156 = call "SR52XX Configure Output Channels - Slope, TC and Dyn Reserve"("VISA session (for class)"=w288, "Time Constant"=w266, "Slope"=w265, "error in (no error)"=w287, "Update"=w283) -> ("VISA session"=w285:refnum<visa-resource-name>)  [unwired: 11 in, 3 out]
              n157 = Bundle By Name(cluster=w279, "slope"=w265, "Input Mode"=w273, "time constant"=w266, "display type"=w282, "Range"=w269, "Line reject"=w278, "Filter Type"=w277, "Auto freq tuning"=w275, "Filter Frequency (Hz)"=w274, "Auto Sensitivity"=w281, "Auto Measure"=w267, "Auto Phase"=w281) -> (w280:T1)
              n158 = local write "Lockin panel"(w280) -> ()
            }
            frame #3 {
              # "Loop Step/Wait/Measure Sequence"
              n159 = To Word Integer(number=w304) -> (16bit integer=w303:i16)
              n160 = for {
                N: w303 -> [_]
                tunnel: w306 -> [w315]
                tunnel: w305 -> [w314]
                tunnel: w302 -> [w313]
                tunnel: w301 -> [w312]
                tunnel: w300 -> [w311]
                tunnel: w299 -> [w310]
                tunnel: w298 -> [w309]
                tunnel: w297 -> [w308]
                tunnel: w296 -> [w307]
                i -> [w316]
                n161 = stacked-sequence {
                  seq-local: [_ _ w332 _ _ _ _ _ _ _ _] -> [_ _ _ _ _ _ w371 w397 _ _ _]
                  seq-local: [_ _ _ _ w338 _ _ _ _ _ _] -> [_ _ _ _ _ _ w375 w393 _ _ _]
                  seq-local: [_ _ _ _ _ _ w370 _ _ _ _] -> [_ _ _ _ _ _ _ w387 _ _ _]
                  seq-local: [_ _ _ _ _ w355 _ _ _ _ _] -> [_ _ _ _ _ _ w376 w385 _ _ _]
                  seq-local: [_ _ _ _ _ _ _ _ w402 _ _] -> [_ _ _ _ _ _ _ _ _ w431 _]
                  seq-local: [_ _ _ _ _ _ _ _ w401 _ _] -> [_ _ _ _ _ _ _ _ _ w430 _]
                  tunnel: w316 -> [_ _ _ _ _ _ w382 _ _ _ _]
                  tunnel: w315 -> [_ _ _ _ _ _ _ _ _ _ w449]
                  tunnel: w314 -> [_ _ _ _ _ _ _ _ _ _ w448]
                  tunnel: w313 -> [w317 _ w333 _ w339 _ _ _ _ _ _]
                  tunnel: w312 -> [_ _ _ _ _ _ w374 _ _ _ _]
                  tunnel: w311 -> [_ _ _ _ _ _ _ w391 w406 _ _]
                  tunnel: w310 -> [_ _ _ _ _ _ _ w392 w405 _ _]
                  tunnel: w309 -> [_ _ _ _ _ w356 _ _ _ _ _]
                  tunnel: w308 -> [_ _ _ _ _ _ _ w386 _ w435 _]
                  tunnel: w307 -> [_ w331 _ _ _ _ _ _ _ _ _]
                  frame #0 {
                    n162 = stacked-sequence {
                      tunnel: w317 -> [w318 _ w321 _ w324 _ w327]
                      frame #0 {
                        # "Sets N PERIODS (number of\ncount periods) to 1."
                        n163 = GPIB Write(0:w318, 1:"NP 1", 2:0) -> ()  [unwired: 2 in, 2 out]
                      }
                      frame #1 {
                        n164 = call "Time Delay4"() -> ()  [unwired: 11 in, 1 out]
                      }
                      frame #2 {
                        # "Clears the counters, sets the SRQ."
                        n165 = GPIB Write(0:w321, 1:"CR;SV 4;", 2:3) -> ()  [unwired: 2 in, 2 out]
                      }
                      frame #3 {
                        n166 = call "Time Delay5"() -> ()  [unwired: 11 in, 1 out]
                      }
                      frame #4 {
                        # "Starts a new scan and returns the  \nA counter buffered data point\nat the end of the count period."
                        n167 = GPIB Write(0:w324, 1:"FA", 2:3) -> ()  [unwired: 2 in, 2 out]
                      }
                      frame #5 {
                        n168 = call "Time Delay6"() -> ()  [unwired: 11 in, 1 out]
                      }
                      frame #6 {
                        # "Disables the timeout function\nand writes the polled \nSRQ values to the front panel.\n(Not clear this step is necessary.)"
                        n169 = Wait for GPIB RQS(3:0, 4:w327) -> ()  [unwired: 1 in, 2 out]
                      }
                    }
                  }
                  frame #1 {
                    # "Waits before reading the data.\nUser should set the wait time to the Tpreset time."
                    n170 = Multiply(x=w331, y=1000.0) -> (x*y=w329:dbl)
                    n171 = Wait (ms)(milliseconds to wait=w329) -> ()  [unwired: 1 out]
                  }
                  frame #2 {
                    # "Read A counter output"
                    n172 = GPIB Read(0:w333, 1:20, 2:0) -> (5:w334:string)  [unwired: 2 in, 2 out]
                    n173 = Fract/Exp String To Number(use system decimal point (T)=FALSE, string=w334) -> (number=w332:dbl)  [unwired: 2 in, 1 out]
                    "counter A" <- w332
                  }
                  frame #3 {
                    n174 = call "Time Delay"() -> ()  [unwired: 11 in, 1 out]
                  }
                  frame #4 {
                    n175 = stacked-sequence {
                      tunnel: w339 -> [w340 _ w344 _]
                      tunnel: [_ _ w343 _] -> w338
                      frame #0 {
                        # "Dumps counter B buffered data point."
                        n176 = GPIB Write(0:w340, 1:"EB", 2:0) -> ()  [unwired: 2 in, 2 out]
                      }
                      frame #1 {
                        n177 = call "Time Delay2"() -> ()  [unwired: 11 in, 1 out]
                      }
                      frame #2 {
                        # "Reads the B counter output"
                        n178 = GPIB Read(0:w344, 1:20, 2:0) -> (5:w345:string)  [unwired: 2 in, 2 out]
                        n179 = Fract/Exp String To Number(use system decimal point (T)=FALSE, string=w345) -> (number=w343:dbl)  [unwired: 2 in, 1 out]
                      }
                      frame #3 {
                        n180 = call "Time Delay3"() -> ()  [unwired: 11 in, 1 out]
                      }
                    }
                    "counter B" <- w338
                  }
                  frame #5 {
                    # "Read Lockin Output"
                    n181 = local read "Lockin panel"() -> (w354:T1)
                    n182 = Unbundle By Name(w354) -> ("slope"=w353:i32, "Input Mode"=w352:i32, "time constant"=w351:i32, "display type"=w350:i32, "Range"=w349:i32)
                    n183 = call "SR5209 Read Output"("VISA session (for class)"=w356, "Input Mode"=w352, "Time Constant"=w351, "Display Type"=w350, "Range"=w349, "Slope"=w353) -> ("Output (FP)"=w355:dbl)  [unwired: 5 in, 8 out]
                    "lockin" <- w355
                  }
                  frame #6 {
                    w360 = "\t"
                    # "lockin"
                    # "counter B"
                    # "counter A"
                    # "wavelength"
                    # "Write to Temp File"
                    # "Current Wavelength"
                    n184 = Get Date/Time In Seconds() -> (seconds since 1Jan1904=w373:timestamp)
                    n185 = To Double Precision Float(number=w373) -> (double precision float=w372:dbl)
                    n186 = local read "Step Size (nm) (sweep2)"() -> (w381:dbl)
                    n187 = local read "Initial Wavelength (sweep2)"() -> (w383:dbl)
                    n188 = Concatenate Strings(w360, "Green Filter in = 1", w360, "532 power", w360, "raster settings\nxV xHz yV yHz", w360, "note", w360, "\r\n") -> (w364:string)
                    n189 = Multiply(x=w382, y=w381) -> (x*y=w380:dbl)
                    n190 = Add(x=w383, y=w380) -> (x+y=w370:dbl)
                    "wavelength" <- w370
                    n191 = Build Array(w370, w371, w375, w376, w372) -> (w377:dbl[])
                    n192 = Array To Spreadsheet String(array=w377, 3:"%#.10g" ("format string")) -> (spreadsheet string=w361:string)  [unwired: 1 in]
                    n193 = String Length(string=w361) -> (length=w359:i32)
                    n194 = Subtract(x=w359, y=2) -> (x-y=w362:i32)
                    n195 = String Subset(string=w361, length (rest)=w362) -> (substring=w363:string)  [unwired: 1 in]
                    n196 = Concatenate Strings(w363, w364) -> (w365:string)
                    "String" <- w365
                    n197 = call <vilib>:"Write Characters To File.vi"("append to file? (new file:F)"=TRUE, "character string"=w365, "file path (dialog if empty)"=w374) -> ()  [unwired: 2 in, 1 out]
                  }
                  frame #7 {
                    w384 = "%#.10g" ("format string")
                    # "Write to Temp Files for graphing."
                    n198 = Build Array(w387, w393) -> (w395:dbl[])
                    n199 = Build Array(w387, w397) -> (w399:dbl[])
                    n200 = Build Array(w387, w385) -> (w389:dbl[])
                    n201 = Array To Spreadsheet String(array=w395, 3:w384) -> (spreadsheet string=w394:string)  [unwired: 1 in]
                    n202 = Array To Spreadsheet String(array=w399, 3:w384) -> (spreadsheet string=w398:string)  [unwired: 1 in]
                    n203 = Array To Spreadsheet String(array=w389, 3:w384) -> (spreadsheet string=w388:string)  [unwired: 1 in]
                    n204 = call <vilib>:"Write Characters To File.vi"("append to file? (new file:F)"=TRUE, "character string"=w394, "file path (dialog if empty)"=w392) -> ()  [unwired: 2 in, 1 out]
                    n205 = call <vilib>:"Write Characters To File.vi"("append to file? (new file:F)"=TRUE, "character string"=w398, "file path (dialog if empty)"=w391) -> ()  [unwired: 2 in, 1 out]
                    n206 = call <vilib>:"Write Characters To File.vi"("append to file? (new file:F)"=TRUE, "character string"=w388, "file path (dialog if empty)"=w386) -> ()  [unwired: 2 in, 1 out]
                  }
                  frame #8 {
                    # "Counter B graph"
                    # "Counter A graph"
                    # "Reads Temp files and sends to  Graph"
                    n207 = call-poly <vilib>:"Read From Spreadsheet File.vi"("format (%.3f)"="%#.10g" ("format string"), "file path (dialog if empty)"=w405) -> ("all rows"=w413:dbl[][])  [unwired: 5 in, 4 out]
                    n208 = call-poly <vilib>:"Read From Spreadsheet File.vi"("format (%.3f)"="%#.10g" ("format string"), "file path (dialog if empty)"=w406) -> ("all rows"=w416:dbl[][])  [unwired: 5 in, 4 out]
                    n209 = Delete From Array(array=w413, index (col)=0 ("disabled index (col)")) -> (deleted portion=w409:dbl[])  [unwired: 2 in, 1 out]
                    n210 = Delete From Array(array=w416, index (col)=0 ("disabled index (col)")) -> (deleted portion=w408:dbl[])  [unwired: 2 in, 1 out]
                    n211 = Delete From Array(array=w416, index (col)=1 ("disabled index (col)")) -> (deleted portion=w407:dbl[])  [unwired: 2 in, 1 out]
                    n212 = Delete From Array(array=w413, index (col)=1 ("disabled index (col)")) -> (deleted portion=w410:dbl[])  [unwired: 2 in, 1 out]
                    n213 = Bundle "Bundle"("all rows"=w409, "all rows"=w410) -> (w402:cluster{"all rows":dbl[], "all rows":dbl[]})  [unwired: 1 in]
                    n214 = Bundle "Bundle"("all rows"=w408, "all rows"=w407) -> (w401:cluster{"all rows":dbl[], "all rows":dbl[]})  [unwired: 1 in]
                    n215 = Build Array(w401, w402) -> (→"Counter Graph":cluster{"all rows":dbl[], "all rows":dbl[]}[])
                  }
                  frame #9 {
                    # "lockin graph"
                    n216 = Unbundle(w430) -> ("all rows"=w420:dbl[], "all rows"=w422:dbl[])
                    n217 = Unbundle(w431) -> ("all rows"=w423:dbl[], "all rows"=w425:dbl[])
                    n218 = call-poly <vilib>:"Read From Spreadsheet File.vi"("format (%.3f)"="%#.10g" ("format string"), "file path (dialog if empty)"=w435) -> ("all rows"=w419:dbl[][])  [unwired: 5 in, 4 out]
                    n219 = Delete From Array(array=w419, index (col)=0 ("disabled index (col)")) -> (deleted portion=w428:dbl[])  [unwired: 2 in, 1 out]
                    n220 = Delete From Array(array=w419, index (col)=1 ("disabled index (col)")) -> (deleted portion=w418:dbl[])  [unwired: 2 in, 1 out]
                    n221 = for {
                      tunnel: w425 -> [w441] mode=indexing
                      tunnel: w422 -> [w440] mode=indexing
                      tunnel: w418 -> [w442] mode=indexing
                      tunnel: [w439] -> w421 mode=indexing
                      tunnel: [w438] -> w424 mode=indexing
                      n222 = Divide(x=w440, y=w442) -> (x/y=w439:dbl)
                      n223 = Divide(x=w441, y=w442) -> (x/y=w438:dbl)
                    }
                    n224 = Bundle "Bundle"("all rows"=w428, "all rows"=w418) -> (w432:cluster{"all rows":dbl[], "all rows":dbl[]})  [unwired: 1 in]
                    n225 = Build Array(w432) -> (→"Lockin Graph":cluster{"all rows":dbl[], "all rows":dbl[]}[])
                    n226 = Bundle "Bundle"("all rows"=w423, w424) -> (w429:cluster{"all rows":dbl[], dbl[]})  [unwired: 1 in]
                    n227 = Bundle "Bundle"("all rows"=w420, w421) -> (w427:cluster{"all rows":dbl[], dbl[]})  [unwired: 1 in]
                    n228 = Build Array(w427, w429) -> (→"Lockin corrected counter graoh":cluster{"all rows":dbl[], dbl[]}[])
                  }
                  frame #10 {
                    # "Step to Next Wavelength"
                    n229 = local read "Step Size (nm) (sweep2)"() -> (w447:dbl)
                    n230 = Multiply(x=w447, y=50.0) -> (x*y=w445:dbl)
                    n231 = To Long Integer(number=w445) -> (32bit integer=w443:i32)
                    n232 = call "monostepgf.vi"("Wait Between Steps(ms)"=u32 8, "Steps"=w443, "Direction"=w448, "address"=w449) -> ()
                  }
                }
              }
            }
            frame #4 {
              # "Set Final Location"
              n233 = local read "Step Size (nm) (sweep2)"() -> (w466:dbl)
              n234 = local read "Initial Wavelength (sweep2)"() -> (w467:dbl)
              n235 = local read "Start Wavelength"() -> (w451:dbl)
              n236 = Multiply(x=w464, y=w466) -> (x*y=w465:dbl)
              n237 = Add(x=w467, y=w465) -> (x+y=w452:dbl)
              n238 = Subtract(x=w451, y=w452) -> (x-y=w455:dbl)
              n239 = Multiply(x=w455, y=50.0) -> (x*y=w462:dbl)
              n240 = Round Toward -Infinity(1:w462) -> (0:w457:dbl)
              n241 = Greater Or Equal To 0?(x=w455) -> (x >= 0?=w454:bool)
              n242 = Absolute Value(x=w457) -> (abs(x)=w458:dbl)
              n243 = To Long Integer(number=w458) -> (32bit integer=w456:i32)
              n244 = Select(t="up", s=w454, f="down") -> (s? t:f=w459:string)
              n245 = call "monostepgf.vi"("Wait Between Steps(ms)"=u32 8, "Steps"=w456, "Direction"=w459, "address"=w450) -> ()
            }
          }
          n246 = Less?(x=w214, y=250.0) -> (x < y?=w225:bool)
          n247 = Greater?(x=w214, y=800.0) -> (0:w224:bool)
          n248 = Less?(x=w215, y=250.0) -> (x < y?=w221:bool)
          n249 = Greater?(x=w215, y=800.0) -> (0:w220:bool)
          n250 = Or(x=w225, y=w224) -> (x .or. y?=w219:bool)
          n251 = Or(x=w221, y=w220) -> (x .or. y?=w218:bool)
          n252 = Stop(stop? (T)=w219) -> ()
          n253 = Stop(stop? (T)=w218) -> ()
        }
      }
      n254 = local write "Lockin panel"("Lockin panel") -> ()
      n255 = Or(x=w20, y=w19) -> (x .or. y?=→"Wavelength Range Warning":bool)
    }
    frame #1 {
      # "Save Data to File"
      n256 = Two Button Dialog(message="Would you like to save the graph?", 1:"Don't Save" ("F button name (\"Cancel\")"), 2:"Save" ("T button name (\"OK\")")) -> (T button?=w469:bool)
      n257 = case shown="False" w469 {
        tunnel: w468 -> [_ w473]
        frame False {
        }
        frame True {
          n258 = stacked-sequence {
            seq-local: [w475 _] -> [_ w477]
            tunnel: w473 -> [w474 _]
            frame #0 {
              n259 = call-poly <vilib>:"Read From Spreadsheet File.vi"("format (%.3f)"="%e", "file path (dialog if empty)"=w474) -> ("all rows"=w475:dbl[][])  [unwired: 5 in, 4 out]
            }
            frame #1 {
              n260 = call-poly <vilib>:"Write To Spreadsheet File.vi"("format (%.3f)"="%e", "2D data"=w477) -> ()  [unwired: 6 in, 1 out]
            }
          }
        }
      }
    }
  }
